vi "FMV - click on close.vi"(8 "error in (no error)":errorcluster) -> (0 "error out":errorcluster)   [LabVIEW 2020, in "ui-testing.lvlib"]
uses:
  ui-testing.lvlib
  User32.dll
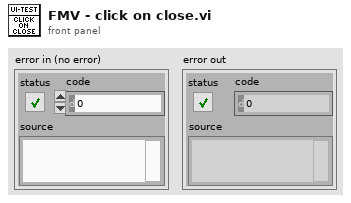
[diagram p1: front panel]
types:
  T1 = typedef "LVRectTypeDef.ctl" = cluster{"Left":i16, "Top":i16, "Right":i16, "Bottom":i16}
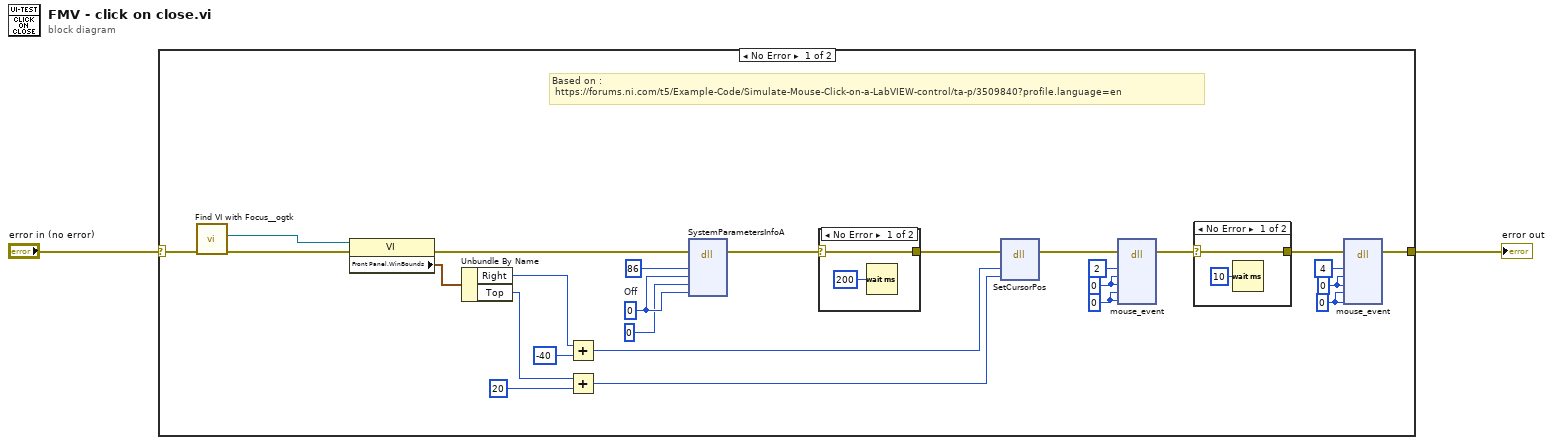
[diagram p0: block diagram]
diagram:
  n1 = case shown="No Error" "error in (no error)" {
    selector: "error in (no error)" -> [w5 w35]
    tunnel: [w14 w35] -> w2
    frame No Error {
      w26 = 0 ("dwExtraInfo")
      w27 = u32 0 ("dwExtraInfo")
      w25 = 0 ("dwExtraInfo")
      w24 = u32 0 ("dwExtraInfo")
      w22 = u32 0  # Off
      # "Based on :\n https://forums.ni.com/t5/Example-Code/Simulate-Mouse-Click-on-a-LabVIEW-control/ta-p/3509840?profile.language=en"
      n2 = call <userlib>:"Find VI with Focus__ogtk.vi"("error in"=w5) -> ("error out"=w4:errorcluster, "VI with Focus"=w3:refnum<vi>)  [unwired: 6 in, 3 out]
      n3 = property class="VI"(reference=w3, error in=w4) -> (error out=w13:errorcluster, "Front Panel.WinBounds"=w10:T1)  [unwired: 1 out]
      n4 = Unbundle By Name(w10) -> ("Right"=w9:i16, "Top"=w8:i16)
      n5 = Add(x=w9, y=i16 -40 ("value")) -> (x+y=w7:i16)
      n6 = Add(x=w8, y=i16 20 ("value")) -> (x+y=w6:i16)
      n7 = dll-call lib="User32.dll" fn="SystemParametersInfoA" label="Terminate power-off mode"(error in=w13, "uiAction"=u32 86 ("SPI_GETPOWEROFFACTIVE"), "uiParam"=w22, "pvParam"=0, "fWinIni"=w22) -> (error out=w19:errorcluster)  [unwired: 7 in, 1 out]
      n8 = case shown="No Error" w19 {
        selector: w19 -> [w32 w34]
        tunnel: [w32 w34] -> w18
        frame No Error {
          n9 = Wait (ms)(milliseconds to wait=u32 200) -> ()  [unwired: 1 out]
        }
        frame Error {
        }
      }
      n10 = dll-call lib="User32.dll" fn="SetCursorPos" label="Move mouse"(error in=w18, "dx"=w7, "dy"=w6) -> (error out=w17:errorcluster)  [unwired: 5 in, 1 out]
      n11 = dll-call lib="User32.dll" fn="mouse_event" label="Click"(error in=w17, "dwFlags"=2, "dx"=w25, "dy"=w25, "dwData"=w24, "dwExtraInfo"=w24) -> (error out=w16:errorcluster)  [unwired: 8 in, 1 out]
      n12 = case shown="No Error" w16 {
        selector: w16 -> [w29 w31]
        tunnel: [w29 w31] -> w15
        frame No Error {
          n13 = Wait (ms)(milliseconds to wait=u32 10) -> ()  [unwired: 1 out]
        }
        frame Error {
        }
      }
      n14 = dll-call lib="User32.dll" fn="mouse_event" label="Release"(error in=w15, "dwFlags"=4, "dx"=w26, "dy"=w26, "dwData"=w27, "dwExtraInfo"=w27) -> (error out=w14:errorcluster)  [unwired: 8 in, 1 out]
    }
    frame Error {
    }
  }
  "error out" <- w2
